vi "Bar Figure.vi"(8 "error in":errorcluster) -> (0 "error out":errorcluster)   [LabVIEW 2020]
uses:
  <vilib>/Heliosphere Research LLC/Advanced Plotting Toolkit/api_annotations/LabelProperties.ctl
  <vilib>/Heliosphere Research LLC/Advanced Plotting Toolkit/properties/Text.ctl
  <vilib>/Heliosphere Research LLC/Advanced Plotting Toolkit/typedefs/PlotColor.ctl
  <vilib>/Heliosphere Research LLC/Advanced Plotting Toolkit/properties/Text_FontSize.ctl
  <vilib>/Heliosphere Research LLC/Advanced Plotting Toolkit/properties/Text_FontStyle.ctl
  <vilib>/Heliosphere Research LLC/Advanced Plotting Toolkit/api_plotting/ErrorbarProperties.ctl
  <vilib>/Heliosphere Research LLC/Advanced Plotting Toolkit/properties/Display.ctl
  <vilib>/Heliosphere Research LLC/Advanced Plotting Toolkit/api_plotting/BarProperties.ctl
  <vilib>/Heliosphere Research LLC/Advanced Plotting Toolkit/properties/Line.ctl
  <vilib>/Heliosphere Research LLC/Advanced Plotting Toolkit/properties/Line_Style.ctl
  <userlib>/_OpenG.lib/array/array.llb/Empty 2D Array (DBL)__ogtk.vi
  <vilib>/Heliosphere Research LLC/Advanced Plotting Toolkit/Advanced Plotting Toolkit.lvlib
  <vilib>/Analysis/NI_AALBase.lvlib
panel:
  out "Means":picture
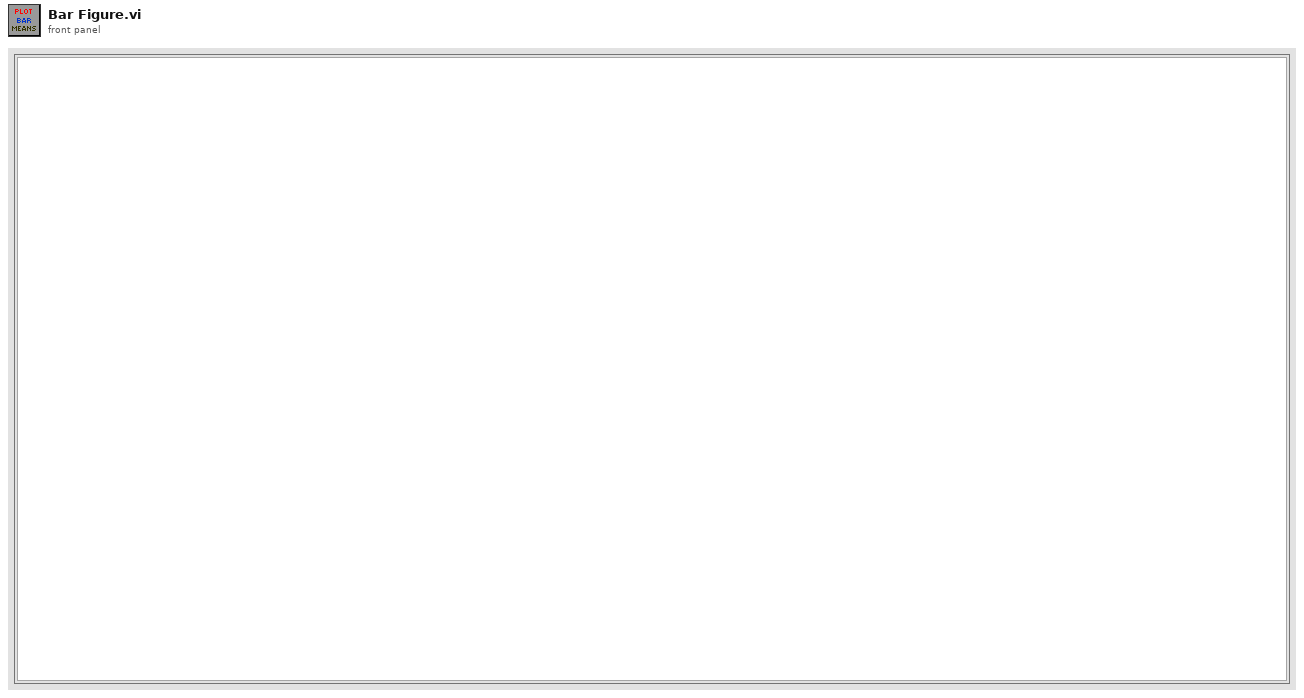
[diagram p1: front panel]
types:
  T1 = typedef "Advanced Plotting Toolkit.lvlib/ErrorbarProperties.ctl" = cluster{"Color":T2, "Line Width":dbl, "Cap Size":dbl, "Display":T3}
  T2 = typedef "Advanced Plotting Toolkit.lvlib/PlotColor.ctl" = u32
  T3 = typedef "Advanced Plotting Toolkit.lvlib/Display.ctl" = cluster{"Alpha":dbl, "Z Order":dbl}
  T4 = typedef "Advanced Plotting Toolkit.lvlib/LabelProperties.ctl" = cluster{"Text":T5}
  T5 = typedef "Advanced Plotting Toolkit.lvlib/Text.ctl" = cluster{"Color":T2, "Background Color":T2, "Font Size (points)":T6, "Font Style":T7, "Rotation Angle":dbl}
  T6 = typedef "Advanced Plotting Toolkit.lvlib/Text_FontSize.ctl" = i32
  T7 = typedef "Advanced Plotting Toolkit.lvlib/Text_FontStyle.ctl" = enum16{"Automatic", "Normal", "Italic", "Bold"}
  T8 = typedef "Advanced Plotting Toolkit.lvlib/BarProperties.ctl" = cluster{"Bar Color":T2, "Line":T9, "Display":T3}
  T9 = typedef "Advanced Plotting Toolkit.lvlib/Line.ctl" = cluster{"Style":T10, "Color":T2, "Width":sgl}
  T10 = typedef "Advanced Plotting Toolkit.lvlib/Line_Style.ctl" = enum16{"Automatic", "Solid", "Dashed", "Dotted", "Dash-dot", "Invisible"}
  T11 = typedef "Advanced Plotting Toolkit.lvlib/PlotID.ctl" = i32
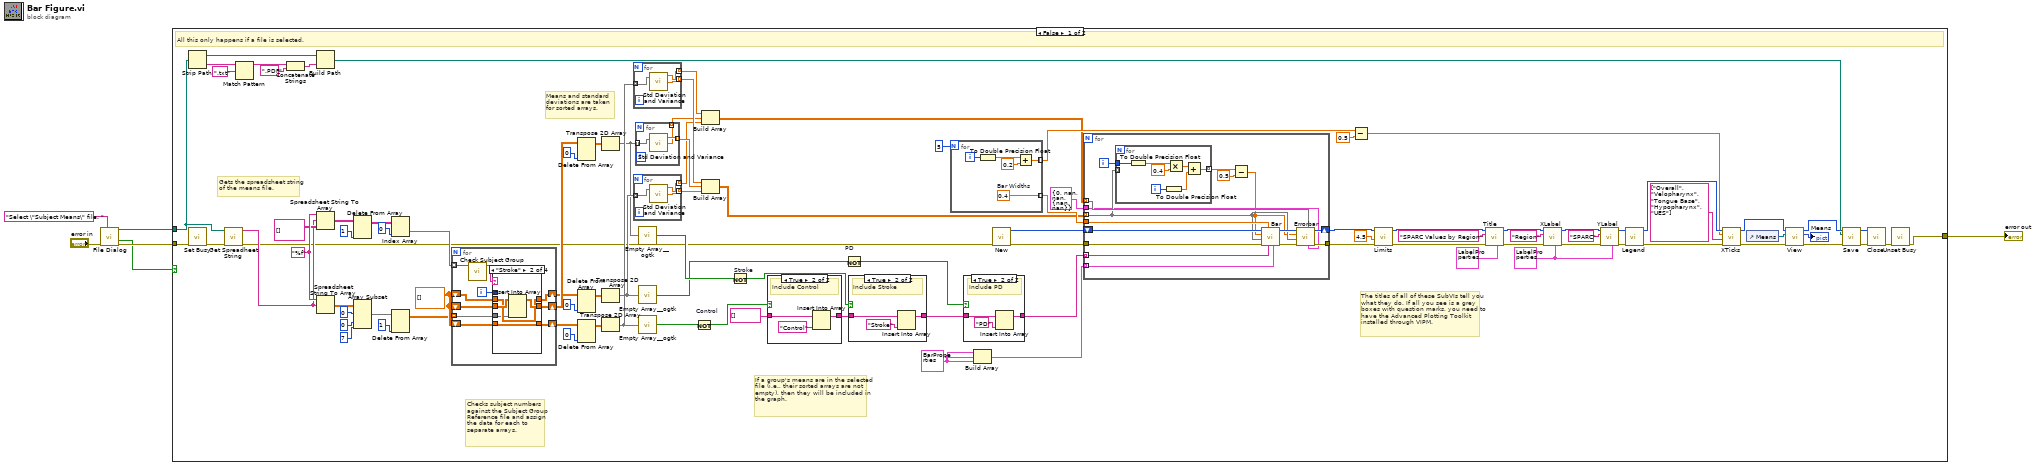
[diagram p0: block diagram]
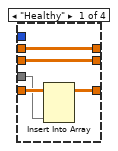
[diagram p5: hidden frame]
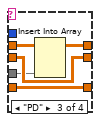
[diagram p6: hidden frame]
diagram:
  n1 = call "File Dialog"("prompt"="Select \"Subject Means\" file. " ("default name"), "error in"="error in") -> ("selected path"=w4:path, "cancelled"=w2:bool, "error out"=w5:errorcluster)  [unwired: 10 in, 1 out]
  n2 = case shown="False" w2 {
    tunnel: w5 -> [w56 w180]
    tunnel: w4 -> [w11 _]
    tunnel: [w7 w180] -> w3
    frame False {
      w47 = dbl[][] []
      w41 = T8 {"Bar Color"=2147483647, "Line"={"Style"=enum."Automatic", "Color"=2147483647, "Width"=nan}, "Display"={"Alpha"=nan, "Z Order"=nan}} ("Properties 2")
      w72 = T4 {"Text"={"Color"=2147483647, "Background Color"=2147483647, "Font Size (points)"=-4, "Font Style"=enum."Bold", "Rotation Angle"=nan}} ("Properties")
      w54 = "%f" ("format string")
      # "The titles of all of these SubVIs tell you what they do. If all you see is a grey boxes with question marks, you need to have the Advanced Plotting Toolkit installed through VIPM."
      # "Means and standard deviations are taken for sorted arrays."
      # "If a group's means are in the selected file (i.e., their sorted arrays are not empty), then they will be included in the graph."
      # "Checks subject numbers against the Subject Group Reference file and assign the data for each to separate arrays."
      # "Gets the spreadsheet string of the means file."
      # "All this only happens if a file is selected."
      n3 = Strip Path(path=w11) -> (stripped path=w63:path, name=w62:string)
      n4 = call <vilib>:"Set Busy.vi"("error in (no error)"=w56) -> ("error out"=w8:errorcluster)  [unwired: 9 in, 1 out]
      n5 = call "Get Spreadheet String.vi"("error in (no error)"=w8, "File Path"=w11) -> ("error out"=w9:errorcluster, "Spreadsheet String"=w10:string)  [unwired: 8 in]
      n6 = Match Pattern(string=w62, regular expression=".txt") -> (before substring=w59:string)  [unwired: 1 in, 3 out]
      n7 = Concatenate Strings(w59, ".PDF" ("string")) -> (w60:string)
      n8 = Build Path(base path=w63, name or relative path=w60) -> (appended path=w57:path)
      n9 = Spreadsheet String To Array(format string=w54, spreadsheet string=w10, array type (2D Dbl)=string[][] []) -> (array=w45:string[][])  [unwired: 1 in]
      n10 = Spreadsheet String To Array(format string=w54, spreadsheet string=w10) -> (array=w34:dbl[][])  [unwired: 2 in]
      n11 = Delete From Array(array=w45, index (col)=1 ("disabled index (col)")) -> (array with subset deleted=w44:string[][])  [unwired: 2 in, 1 out]
      n12 = Array Subset(array=w34, index (row)=0 ("index"), index (col)=0 ("index"), length (col)=7 ("length")) -> (w33:dbl[][])  [unwired: 1 in]
      n13 = Index Array(array=w44, index (col)=0 ("disabled index (col)")) -> (element=w49:string[])  [unwired: 1 in]
      n14 = Delete From Array(array=w33, index (col)=1 ("disabled index (col)")) -> (array with subset deleted=w46:dbl[][])  [unwired: 2 in, 1 out]
      n15 = for {
        tunnel: w49 -> [w126] mode=indexing
        shift-right: [w120] -> w35
        shift-left: w47 -> [w121]
        shift-right: [w124] -> w37
        shift-left: w47 -> [w125]
        shift-right: [w122] -> w39
        shift-left: w47 -> [w123]
        tunnel: w46 -> [w118] mode=indexing
        i -> [w119]
        n16 = call "Check Subject Group.vi"("Subject Number"=w126) -> ("Group"=w127:string)  [unwired: 10 in]
        n17 = case shown="\"Stroke\"" w127 {
          tunnel: w119 -> [_ _ _ _]
          tunnel: w125 -> [w130 w137 w140 w143]
          tunnel: [w130 w136 w140 w143] -> w124
          tunnel: w123 -> [w132 w135 w139 w145]
          tunnel: [w131 w135 w139 w145] -> w122
          tunnel: w121 -> [w129 w134 w142 w144]
          tunnel: [w129 w134 w141 w144] -> w120
          tunnel: w118 -> [w128 w133 w138 _]
          frame "Healthy" {
            n18 = Insert Into Array(array=w132, new element=w128) -> (w131:dbl[][])  [unwired: 2 in]
          }
          frame "Stroke" {
            n19 = Insert Into Array(array=w137, new element=w133) -> (w136:dbl[][])  [unwired: 2 in]
          }
          frame "PD" {
            n20 = Insert Into Array(array=w142, new element=w138) -> (w141:dbl[][])  [unwired: 2 in]
          }
          frame Default {
          }
        }
      }
      n21 = Delete From Array(array=w37, index (col)=0) -> (array with subset deleted=w29:dbl[][])  [unwired: 2 in, 1 out]
      n22 = Delete From Array(array=w35, index (col)=0) -> (array with subset deleted=w26:dbl[][])  [unwired: 2 in, 1 out]
      n23 = Delete From Array(array=w39, index (col)=0) -> (array with subset deleted=w28:dbl[][])  [unwired: 2 in, 1 out]
      n24 = Transpose 2D Array(2D array=w29) -> (transposed array=w12:dbl[][])
      n25 = Transpose 2D Array(2D array=w26) -> (transposed array=w20:dbl[][])
      n26 = Transpose 2D Array(2D array=w28) -> (transposed array=w22:dbl[][])
      n27 = for {
        tunnel: w22 -> [w176] mode=indexing
        tunnel: [w175] -> w97 mode=indexing
        tunnel: [w174] -> w52 mode=indexing
        n28 = call <vilib>:"Std Deviation and Variance.vi"("X"=w176) -> ("mean"=w175:dbl, "standard deviation"=w174:dbl)  [unwired: 1 in, 1 out]
      }
      n29 = for {
        tunnel: w20 -> [w117] mode=indexing
        tunnel: [w116] -> w25 mode=indexing
        tunnel: [w115] -> w24 mode=indexing
        n30 = call <vilib>:"Std Deviation and Variance.vi"("X"=w117) -> ("mean"=w116:dbl, "standard deviation"=w115:dbl)  [unwired: 1 in, 1 out]
      }
      n31 = for {
        tunnel: w12 -> [w179] mode=indexing
        tunnel: [w178] -> w98 mode=indexing
        tunnel: [w177] -> w51 mode=indexing
        n32 = call <vilib>:"Std Deviation and Variance.vi"("X"=w179) -> ("mean"=w178:dbl, "standard deviation"=w177:dbl)  [unwired: 1 in, 1 out]
      }
      n33 = call-poly <userlib>:"Empty Array__ogtk.vi"("Array"=w12) -> ("Empty Array?"=w27:bool)  [unwired: 8 in]
      n34 = call-poly <userlib>:"Empty Array__ogtk.vi"("Array"=w20) -> ("Empty Array?"=w21:bool)  [unwired: 8 in]
      n35 = call-poly <userlib>:"Empty Array__ogtk.vi"("Array"=w22) -> ("Empty Array?"=w23:bool)  [unwired: 8 in]
      n36 = Not "Control"(x=w23) -> (.not. x?=w18:bool)
      n37 = Build Array(w52, w51, w24) -> (w50:dbl[][])
      n38 = Build Array(w97, w98, w25) -> (w93:dbl[][])
      n39 = Not "Stroke"(x=w27) -> (.not. x?=w17:bool)
      n40 = case shown="True" w18 {
        tunnel: string[] [] -> [w111 w114]
        tunnel: [w111 w113] -> w15
        frame False {
        }
        frame True {
          # "Include Control"
          n41 = Insert Into Array(array=w114, new element="Control" ("new element/subarray")) -> (w113:string[])  [unwired: 1 in]
        }
      }
      n42 = Not "PD"(x=w21) -> (.not. x?=w16:bool)
      n43 = case shown="True" w17 {
        tunnel: w15 -> [w107 w110]
        tunnel: [w107 w109] -> w14
        frame False {
        }
        frame True {
          # "Include Stroke"
          n44 = Insert Into Array(array=w110, new element="Stroke" ("new element/subarray")) -> (w109:string[])  [unwired: 1 in]
        }
      }
      n45 = for {
        N: 5 -> [_]
        tunnel: [w146] -> w89 mode=indexing
        tunnel: [w149] -> w95 mode=indexing
        i -> [w150]
        w149 = 0.4  # Bar Widths
        n46 = To Double Precision Float(number=w150) -> (double precision float=w147:dbl)
        n47 = Add(x=w147, y=0.2) -> (x+y=w146:dbl)
      }
      n48 = case shown="True" w16 {
        tunnel: w14 -> [w103 w105]
        tunnel: [w103 w106] -> w13
        frame False {
        }
        frame True {
          # "Include PD"
          n49 = Insert Into Array(array=w105, new element="PD" ("new element/subarray")) -> (w106:string[])  [unwired: 1 in]
        }
      }
      n50 = Build Array(w41, w41, w41) -> (w71:T8[])
      n51 = call <vilib>:"New.vi"("error in (no error)"=w9) -> ("error out"=w102:errorcluster, "Plot ID"=w101:T11)  [unwired: 9 in]
      n52 = for {
        tunnel: w102 -> [w165]
        shift-right: [w156] -> w79
        shift-left: w101 -> [w166]
        tunnel: [w155] -> w78
        tunnel: w93 -> [w153] mode=indexing
        tunnel: w95 -> [w163]
        tunnel: w13 -> [w162] mode=indexing
        tunnel: w71 -> [w159] mode=indexing
        tunnel: w50 -> [w158] mode=indexing
        tunnel: T1 {"Color"=0, "Line Width"=nan, "Cap Size"=nan, "Display"={"Alpha"=nan, "Z Order"=nan}} ("Error Bar Props") -> [w152]
        i -> [w164]
        n53 = for {
          tunnel: w164 -> [w173]
          tunnel: w153 -> [_] mode=indexing
          tunnel: [w167] -> w161 mode=indexing
          i -> [w169]
          n54 = To Double Precision Float(number=w173) -> (double precision float=w172:dbl)
          n55 = To Double Precision Float(number=w169) -> (double precision float=w168:dbl)
          n56 = Multiply(x=w172, y=0.4) -> (x*y=w170:dbl)
          n57 = Add(x=w170, y=w168) -> (x+y=w167:dbl)
        }
        n58 = Subtract(x=w161, y=0.5) -> (x-y=w151:dbl[])
        n59 = call <vilib>:"Bar.vi"("Properties"=w159, "Legend Title"=w162, "Bar Widths"=w163, "error in (no error)"=w165, "Bar Lengths"=w153, "X Coordinates"=w151, "Plot ID"=w166) -> ("error out"=w154:errorcluster, "Plot ID Out"=w157:T11)  [unwired: 3 in]
        n60 = call <vilib>:"Errorbar.vi"("Properties"=w152, "Y Errors"=w158, "error in (no error)"=w154, "Y Data"=w153, "X Data"=w151, "Plot ID"=w157) -> ("error out"=w155:errorcluster, "Plot ID out"=w156:T11)  [unwired: 4 in]
      }
      n61 = Subtract(x=w89, y=0.5) -> (x-y=w88:dbl[])
      n62 = call <vilib>:"Limits.vi"("error in (no error)"=w78, "X Max"=4.5, "Plot ID"=w79) -> ("error out"=w80:errorcluster, "Plot ID Out"=w81:T11)  [unwired: 7 in]
      n63 = call <vilib>:"Title.vi"("Properties"=T4 {"Text"={"Color"=2147483647, "Background Color"=2147483647, "Font Size (points)"=-5, "Font Style"=enum."Bold", "Rotation Angle"=nan}}, "error in (no error)"=w80, "Title"="SPARC Values by Region", "Plot ID"=w81) -> ("error out"=w84:errorcluster, "Plot ID out"=w85:T11)  [unwired: 6 in]
      n64 = call <vilib>:"XLabel.vi"("Properties"=w72, "error in (no error)"=w84, "Label"="Region", "Plot ID"=w85) -> ("error out"=w87:errorcluster, "Plot ID out"=w86:T11)  [unwired: 6 in]
      n65 = call <vilib>:"YLabel.vi"("Properties"=w72, "error in (no error)"=w87, "Label"="SPARC", "Plot ID"=w86) -> ("error out"=w82:errorcluster, "Plot ID out"=w83:T11)  [unwired: 6 in]
      n66 = call <vilib>:"Legend.vi"("error in (no error)"=w82, "Plot ID"=w83) -> ("error out"=w91:errorcluster, "Plot ID Out"=w92:T11)  [unwired: 8 in]
      n67 = call <vilib>:"XTicks.vi"("error in (no error)"=w91, "Tick Labels"=string[] ["Overall", "Velopharynx", "Tongue Base", "Hypopharynx", "UES"], "Tick Locations"=w88, "Plot ID"=w92) -> ("error out"=w66:errorcluster, "Plot ID Out"=w65:T11)  [unwired: 6 in]
      n68 = control-ref of="Means"() -> (w100:refnum<vi>)
      n69 = call <vilib>:"View.vi"("error in (no error)"=w66, "Ref for Sizing"=w100, "Plot ID"=w65) -> ("error out"=w67:errorcluster, "Picture"=→"Means":picture, "Plot ID Out"=w70:T11)  [unwired: 6 in]
      n70 = call <vilib>:"Save.vi"("error in (no error)"=w67, "Path"=w57, "Plot ID In"=w70) -> ("error out"=w68:errorcluster, "Plot ID Out"=w69:T11)  [unwired: 7 in]
      n71 = call <vilib>:"Close.vi"("error in (no error)"=w68, "Plot ID"=w69) -> ("error out"=w55:errorcluster)  [unwired: 9 in]
      n72 = call <vilib>:"Unset Busy.vi"("error in (no error)"=w55) -> ("error out"=w7:errorcluster)  [unwired: 10 in]
    }
    frame True {
      # "Nothing happens if file selection is cancelled"
    }
  }
  "error out" <- w3
